vi "RunInferenceAllOutput.vi"(4 "Introspection Output":T1, 8 "error in (no error)":errorcluster, 9 "inputIndex":i32, 10 "inputBuffer":sgl[](array[numeric]), 11 "session id in":i32) -> (0 "error out":errorcluster, 2 "outputBuffer":sgl[](array[numeric]), 3 "session id out":i32)   [LabVIEW 2017, in "libonnx_wrapper.lvlib"]
doc: "/**\n * @brief Выполнить инференс (предсказание) модели\n * \n * Основная функция для получения предсказания от модели. Принимает входные данные,\n * передаёт их в нейросеть и записывает результат в выходной буфер.\n * \n * @param sessionId [IN] ID сессии\n * @param inputIndex [IN] Индекс входа (обычно 0 для моделей с одним входом)\n * @param inputBuffer [IN] Массив входных данных (тип должен соответствовать GetInputType)\n * @param inputSize [IN] Количество элементов во входном массиве\n * @param outputIndex [IN] Индекс выхода (обычно 0 для моделей с одним выходом)\n * @param outputBuffer [OUT] Массив для записи результатов (должен быть выделен в LabVIEW)\n * @param outputSize [IN] Размер выходного буфера в элементах\n * \n * @return int32: 0 при успешном выполнении инференса\n * @return int32: -1 при ошибке (сессия не загружена, неверные индексы, ошибка ONNX Runtime)\n * \n * @note Входные данные должны быть нормализованы так же, как при обучении модели\n * @note Размер входного массива должен соответствовать произведению всех размерностей shape\n * @note Выходной буфер должен быть достаточного размера (см. GetOutputShapeDim)\n * @note Функция блокирует выполнение до завершения инференса\n * \n * @example\n * // Для модели с входом [1, 10] и выходом [1, 3]:\n * float inputData[10] = {...};\n * float outputData[3];\n * RunInference(sessionId, 0, inputData, 10, 0, outputData, 3);\n */\nint RunInference(int sessionId, int inputIndex, float* inputBuffer, int inputSize, \n int outputIndex, float* outputBuffer, int outputSize);"
uses:
  libonnx_wrapper.lvlib
  TypeDef/IO.ctl
  TypeDef/Introspection.ctl
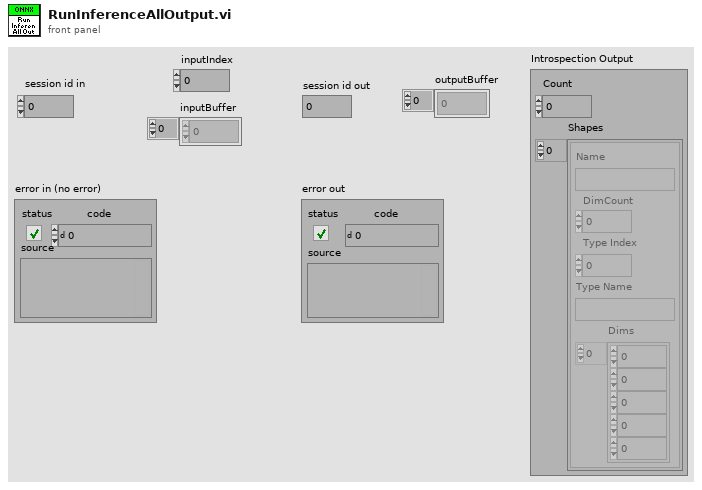
[diagram p1: front panel]
types:
  T1 = typedef "libonnx_wrapper.lvlib/Introspection.ctl" = cluster{"Count":i32, "Shapes":T2[]}
  T2 = typedef "libonnx_wrapper.lvlib/IO.ctl" = cluster{"Name":string, "DimCount":i32, "Type Index":i32, "Type Name":string, "Dims":i64[]}
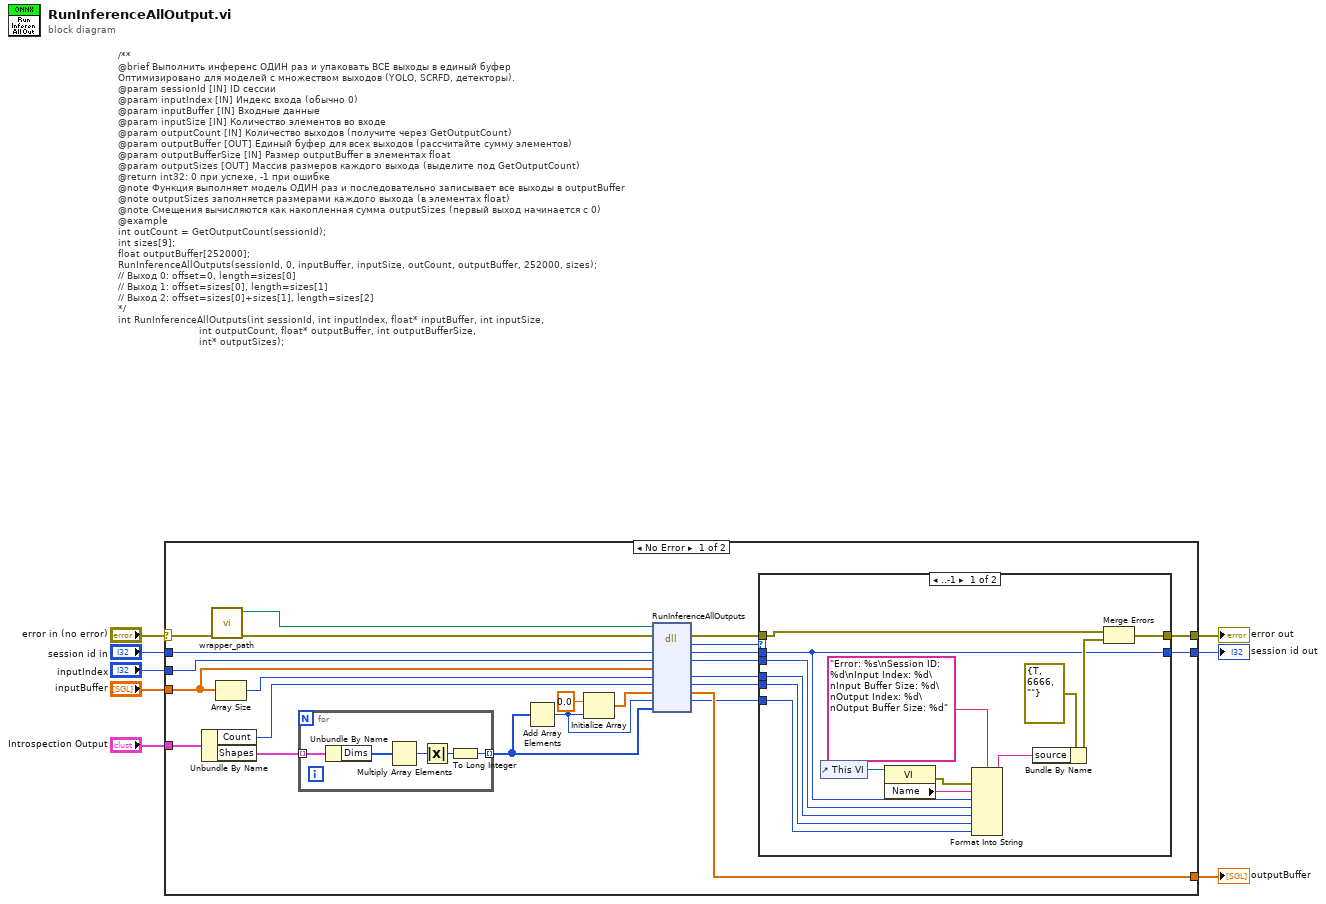
[diagram p0: block diagram]
diagram:
  # "/**\n@brief Выполнить инференс ОДИН раз и упаковать ВСЕ выходы в единый буфер\nОптимизировано для моделей с множеством выходов (YOLO, SCRFD, детекторы).\n@param sessionId [IN] ID сессии\n@param inputIndex [IN] Индекс входа (обычно 0)\n@param inputBuffer [IN] Входные данные\n@param inputSize [IN] Количество элементов во входе\n@param outputCount [IN] Количество выходов (получите через GetOutputCount)\n@param outputBuffer [OUT] Единый буфер для всех выходов (рассчитайте сумму элементов)\n@param outputBufferSize [IN] Размер outputBuffer в элементах float\n@param outputSizes [OUT] Массив размеров каждого выхода (выделите под GetOutputCount)\n@return int32: 0 при успехе, -1 при ошибке\n@note Функция выполняет модель ОДИН раз и последовательно записывает все выходы в outputBuffer\n@note outputSizes заполняется размерами каждого выхода (в элементах float)\n@note Смещения вычисляются как накопленная сумма outputSizes (первый выход начинается с 0)\n@example\nint outCount = GetOutputCount(sessionId);\nint sizes[9];\nfloat outputBuffer[252000];\nRunInferenceAllOutputs(sessionId, 0, inputBuffer, inputSize, outCount, outputBuffer, 252000, sizes);\n// Выход 0: offset=0, length=sizes[0]\n// Выход 1: offset=sizes[0], length=sizes[1]\n// Выход 2: offset=sizes[0]+sizes[1], length=sizes[2]\n*/\nint RunInferenceAllOutputs(int sessionId, int inputIndex, float* inputBuffer, int inputSize,\n                           int outputCount, float* outputBuffer, int outputBufferSize,\n                           int* outputSizes);"
  n1 = case shown="No Error" "error in (no error)" {
    selector: "error in (no error)" -> [w13 w55]
    tunnel: "session id in" -> [w30 w54]
    tunnel: "inputIndex" -> [w29 _]
    tunnel: "inputBuffer" -> [w28 _]
    tunnel: [w24 _] -> w5
    tunnel: "Introspection Output" -> [w23 _]
    tunnel: [w19 w55] -> w3
    tunnel: [w18 w54] -> w2
    frame No Error {
      n2 = Unbundle By Name(w23) -> ("Count"=w12:i32, "Shapes"=w11:T2[])
      n3 = call "wrapper_path.vi"("error in (no error)"=w13) -> ("error out"=w31:errorcluster, "wrapper path"=w32:path)  [unwired: 9 in]
      n4 = Array Size(array=w28) -> (size(s)=w27:i32)
      n5 = for {
        tunnel: [w34] -> w9 mode=indexing
        tunnel: w11 -> [w33] mode=indexing
        n6 = Unbundle By Name(w33) -> ("Dims"=w37:i64[])
        n7 = Multiply Array Elements(1:w37) -> (0:w36:i64)
        n8 = Absolute Value(x=w36) -> (abs(x)=w35:i64)
        n9 = To Long Integer(number=w35) -> (32bit integer=w34:i32)
      }
      n10 = Add Array Elements(numeric array=w9) -> (sum=w10:i32)
      n11 = Initialize Array(sgl 0.0 ("element"), w10) -> (w25:sgl[])
      n12 = dll-call lib="home/ivan/LabVIEWData/ONNX/LabVIEW-ONNX_Runtime/onnx_wrapper/unix64/libonnx_wrapper.so" fn="RunInferenceAllOutputs"(path in=w32, error in=w31, "sessionId"=w30, "inputIndex"=w29, "inputBuffer"=w28, "inputSize"=w27, "outputCount"=w12, "outputBuffer"=w25, "outputBufferSize"=w10, "outputSizes"=w9) -> (error out=w22:errorcluster, "return"=w21:i32, "sessionId"=w20:i32, "inputIndex"=w17:i32, "inputSize"=w16:i32, "outputCount"=w15:i32, "outputBuffer"=w24:sgl[], "outputBufferSize"=w14:i32)  [unwired: 3 in, 1 out]
      n13 = case shown="..-1" w21 {
        tunnel: w22 -> [w42 w53]
        tunnel: [w43 w53] -> w19
        tunnel: w20 -> [w44 w52]
        tunnel: [w44 w52] -> w18
        tunnel: w17 -> [w41 _]
        tunnel: w16 -> [w40 _]
        tunnel: w15 -> [w39 _]
        tunnel: w14 -> [w38 _]
        frame ..-1 {
          n14 = control-ref of="This VI"() -> (w48:refnum<vi>)
          n15 = property class="VI"(reference=w48) -> (error out=w45:errorcluster, "Name"=w47:string)  [unwired: 1 in, 1 out]
          n16 = Format Into String(format string="Error: %s\nSession ID: %d\nInput Index: %d\nInput Buffer Size: %d\nOutput Index: %d\nOutput Buffer Size: %d", error in=w45, w47, w44, w41, w40, w39, w38) -> (resulting string=w49:string)  [unwired: 1 in, 1 out]
          n17 = Bundle By Name(cluster=errorcluster {"status"=TRUE, "code"=6666, "source"=""} ("error out"), "source"=w49) -> (w50:errorcluster)
          n18 = Merge Errors(w42, w50) -> (w43:errorcluster)
        }
        frame 0.. {
        }
      }
    }
    frame Error {
    }
  }
  "error out" <- w3
  "session id out" <- w2
  "outputBuffer" <- w5
